vi "Read Resizable.vi"(9 "FPWindow in":refnum<class "FPWindow.lvclass">) -> (3 "FPWindow out":refnum<class "FPWindow.lvclass">, 4 "Resizable":bool)   [LabVIEW 2014, in "Raspberry Pi Compatible Compiler for LabVIEW.lvlib" / "FPWindow.lvclass"]
uses:
  FPWindow.lvclass
  FPWindow.lvclass/FPWindow.ctl
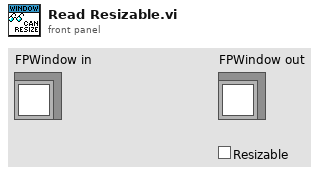
[diagram p1: front panel]
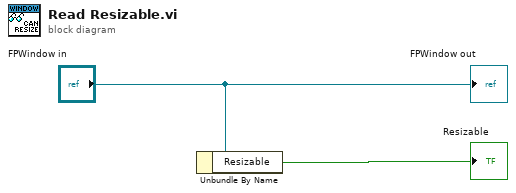
[diagram p0: block diagram]
diagram:
  n1 = Unbundle By Name("FPWindow in") -> ("Resizable"=→"Resizable":bool)
  "FPWindow out" <- "FPWindow in"
